vi "Move Drive Motors.vi"(9 "Pneumatics In":T2={"CompressorDevRef"={"DevStatus"={"status"=FALSE, "code"=0, "source"=""}, "Pneumatics Control Module"=0}, "High and Low Gear DoubleSolenoidDevRef"={"DevStatus"={"status"=FALSE, "code"=0, "source"=""}, "Pneumatics Control Module"=0, "Forward Solenoid Channel"=enum."Invalid", "Reverse Solenoid Channel"=enum."Invalid"}, "PTO SolenoidDevRef"={"DevStatus"={"status"=FALSE, "code"=0, "source"=""}, "Pneumatics Control Module"=0, "Forward Solenoid Channel"=enum."Invalid", "Reverse Solenoid Channel"=enum."Invalid"}, "Hang Pin SolenoidDevRef"={"DevStatus"={"status"=FALSE, "code"=0, "source"=""}, "Pneumatics Control Module"=0, "Forward Solenoid Channel"=enum."Invalid", "Reverse Solenoid Channel"=enum."Invalid"}}, 11 "RobotDriveDevRef":T6={"DevStatus"={"status"=FALSE, "code"=0, "source"=""}, "Motors[]"=[], "Square Inputs"=FALSE, "Max Output"=1.0}) -> (1 "Pneumatics Out":T2={"CompressorDevRef"={"DevStatus"={"status"=FALSE, "code"=0, "source"=""}, "Pneumatics Control Module"=0}, "High and Low Gear DoubleSolenoidDevRef"={"DevStatus"={"status"=FALSE, "code"=0, "source"=""}, "Pneumatics Control Module"=0, "Forward Solenoid Channel"=enum."Invalid", "Reverse Solenoid Channel"=enum."Invalid"}, "PTO SolenoidDevRef"={"DevStatus"={"status"=FALSE, "code"=0, "source"=""}, "Pneumatics Control Module"=0, "Forward Solenoid Channel"=enum."Invalid", "Reverse Solenoid Channel"=enum."Invalid"}, "Hang Pin SolenoidDevRef"={"DevStatus"={"status"=FALSE, "code"=0, "source"=""}, "Pneumatics Control Module"=0, "Forward Solenoid Channel"=enum."Invalid", "Reverse Solenoid Channel"=enum."Invalid"}}, 3 "RobotDriveDevRef 2":T6={"DevStatus"={"status"=FALSE, "code"=0, "source"=""}, "Motors[]"=[], "Square Inputs"=FALSE, "Max Output"=1.0})   [LabVIEW 2015]
uses:
  <vilib>/Rock Robotics/WPI/RobotDrive/WPI_RobotDriveDevRef.ctl
  <vilib>/Rock Robotics/WPI/MotorControl/WPI_MotorControlDeviceRef.ctl
  <vilib>/Rock Robotics/WPI/MotorControl/WPI_MotorControlType.ctl
  <vilib>/Rock Robotics/SystemInterfaces/DIO/FPGA_DIOPWMChannel.ctl
  <vilib>/Rock Robotics/WPI/PWM/WPI_PWMDeadband.ctl
  <vilib>/Rock Robotics/WPI/CAN/Jaguar/SubVIs/WPI_CANJaguar_ControlMode.ctl
  <vilib>/Rock Robotics/WPI/CAN/TalonSRX/WPI_CANTalonSRX_APIControlMode.ctl
  Pnematics.ctl
  <vilib>/Rock Robotics/WPI/Compressor/WPI_CompressorDevRef.ctl
  <vilib>/Rock Robotics/WPI/Solenoid/WPI_SolenoidDevRef.ctl
  <vilib>/Rock Robotics/WPI/Solenoid/WPI_SolenoidChannel.ctl
  <vilib>/Rock Robotics/WPI/Solenoid/WPI_SolenoidValue.ctl
  Robot Values.vi
  <vilib>/Rock Robotics/WPI/Solenoid/WPI_SolenoidSetEnum.vi
  <vilib>/Rock Robotics/Network Tables/NT Write String.vi
panel:
  in  "Low":T1=enum."Forward"
  in  "High":T1=enum."Reverse"
  in  "Limits":cluster{"\"Upper\"":dbl, "\"Lower\"":dbl}={"\"Upper\""=1.0, "\"Lower\""=0.1}
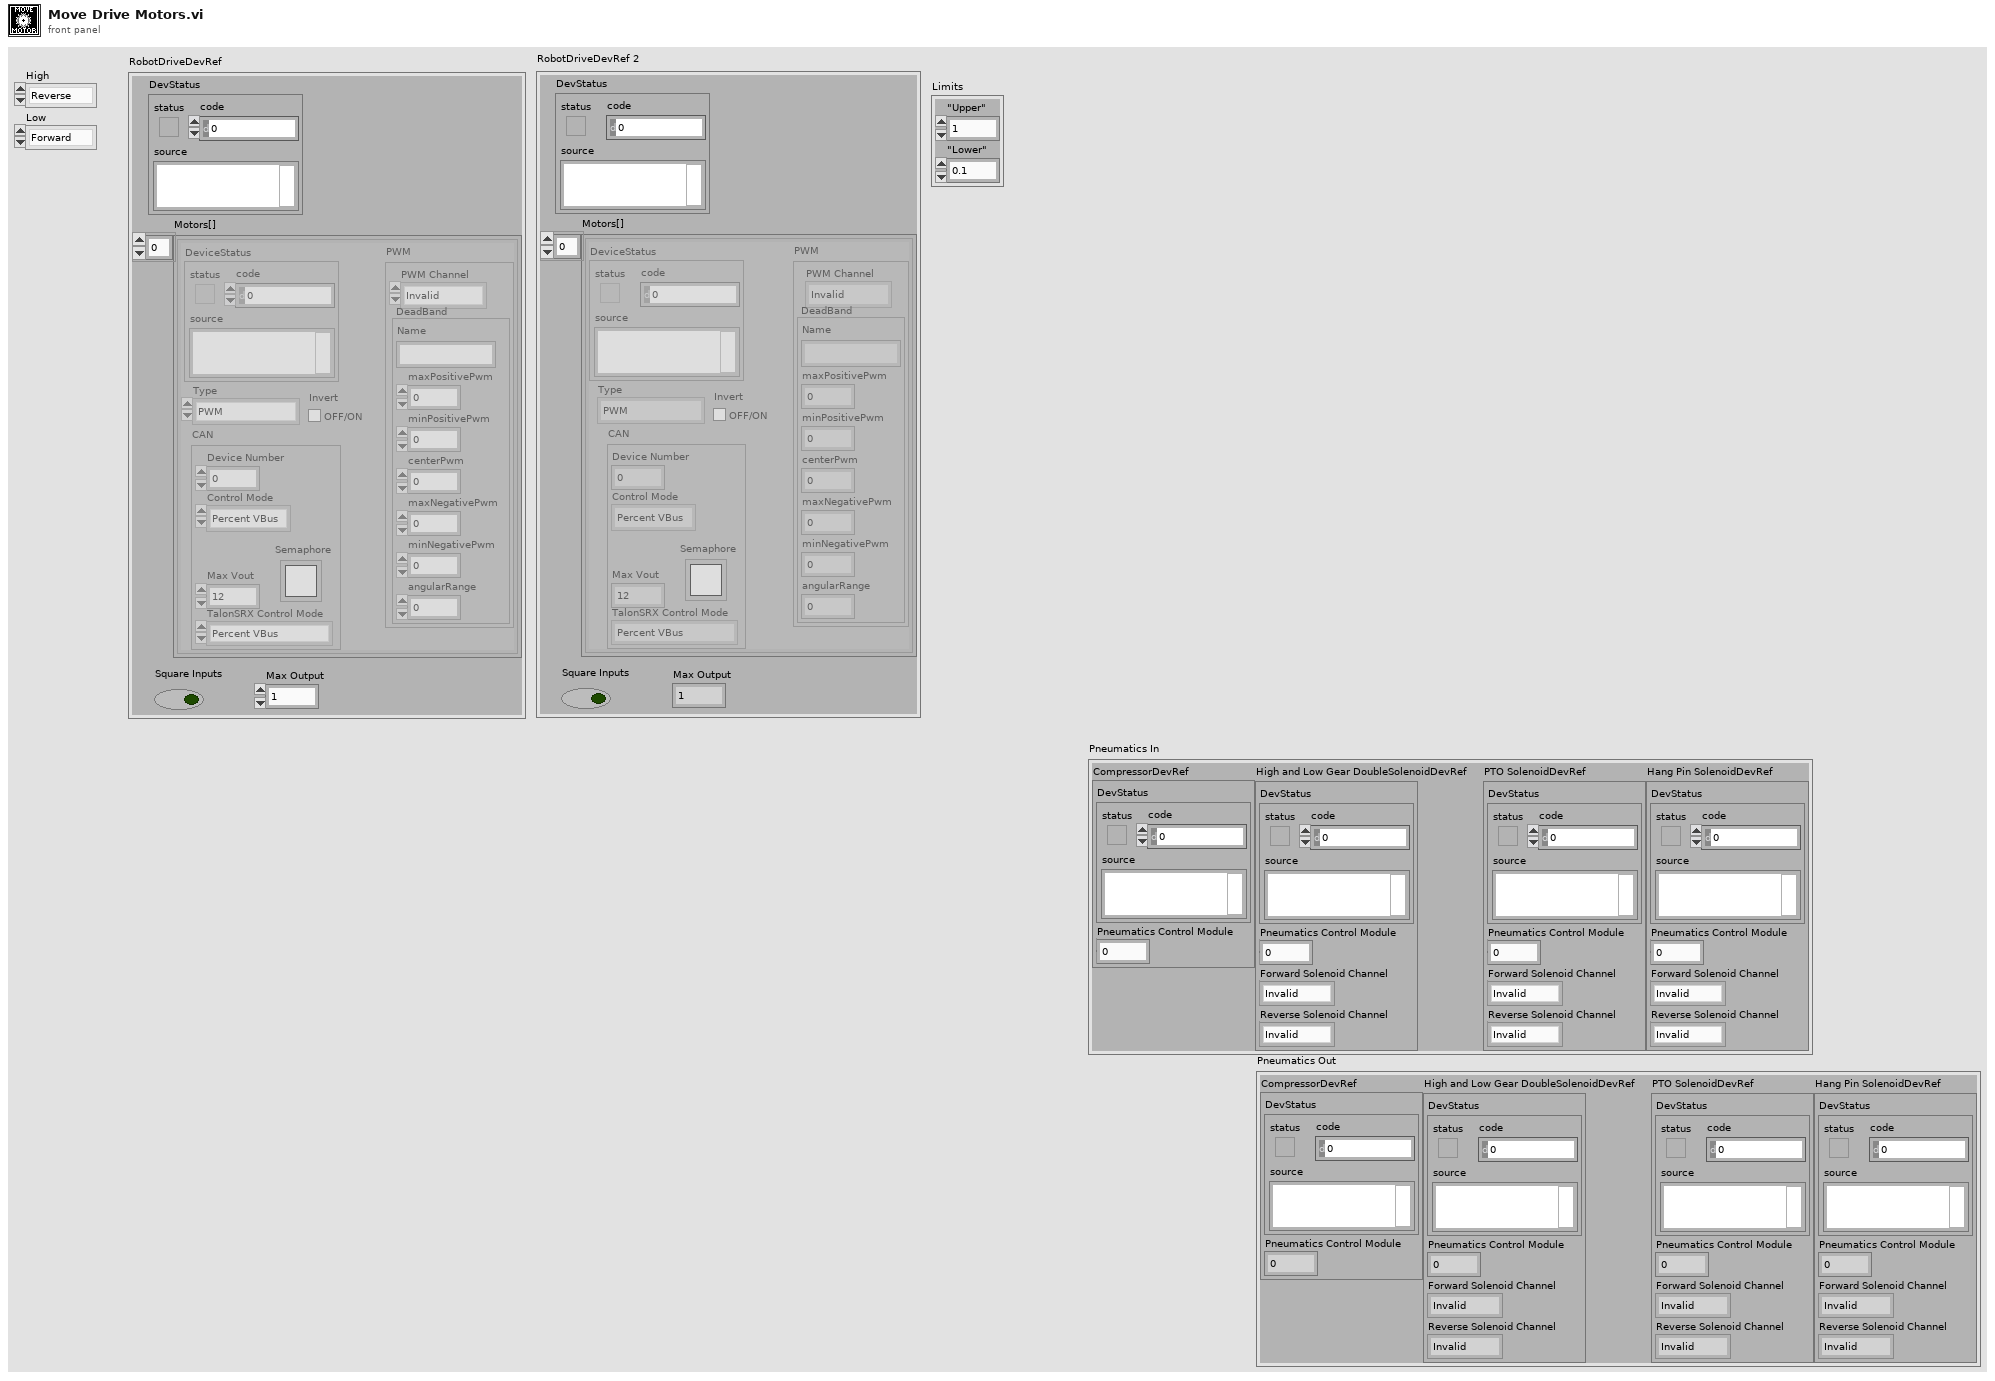
[diagram p1: front panel]
types:
  T1 = typedef "WPI_SolenoidValue.ctl" = enum16{"Off", "On", "Forward", "Reverse"}
  T2 = typedef "Pnematics.ctl" = cluster{"CompressorDevRef":T3, "High and Low Gear DoubleSolenoidDevRef":T4, "PTO SolenoidDevRef":T4, "Hang Pin SolenoidDevRef":T4}
  T3 = typedef "WPI_CompressorDevRef.ctl" = cluster{"DevStatus":errorcluster, "Pneumatics Control Module":u8}
  T4 = typedef "WPI_SolenoidDevRef.ctl" = cluster{"DevStatus":errorcluster, "Pneumatics Control Module":u8, "Forward Solenoid Channel":T5, "Reverse Solenoid Channel":T5}
  T5 = typedef "WPI_SolenoidChannel.ctl" = enum8{"Solenoid 0", "Solenoid 1", "Solenoid 2", "Solenoid 3", "Solenoid 4", "Solenoid 5", "Solenoid 6", "Solenoid 7", "Invalid"}
  T6 = typedef "WPI_RobotDriveDevRef.ctl" = cluster{"DevStatus":errorcluster, "Motors[]":T7[], "Square Inputs":bool, "Max Output":dbl}
  T7 = typedef "WPI_MotorControlDeviceRef.ctl" = cluster{"DeviceStatus":errorcluster, "Type":T8, "PWM":cluster{"PWM Channel":T9, "DeadBand":T10}, "CAN":cluster{"Device Number":u8, "Control Mode":T11, "Semaphore":T12, "Max Vout":dbl, "TalonSRX Control Mode":T13}, "Invert":bool}
  T8 = typedef "WPI_MotorControlType.ctl" = enum16{"PWM", "CAN", "CANTalonSRX"}
  T9 = typedef "FPGA_DIOPWMChannel.ctl" = enum8{"PWM 0", "PWM 1", "PWM 2", "PWM 3", "PWM 4", "PWM 5", "PWM 6", "PWM 7", "PWM 8", "PWM 9", "PWM MXP 0", "PWM MXP 1", "PWM MXP 2", "PWM MXP 3", "PWM MXP 4", "PWM MXP 5", "PWM MXP 6", "PWM MXP 7", "PWM MXP 8", "PWM MXP 9", "Invalid"}
  T10 = typedef "WPI_PWMDeadband.ctl" = cluster{"Name":string, "maxPositivePwm":i32, "minPositivePwm":i32, "centerPwm":i32, "maxNegativePwm":i32, "minNegativePwm":i32, "angularRange":u16}
  T11 = typedef "WPI_CANJaguar_ControlMode.ctl" = enum8{"Percent VBus", "Current", "Speed", "Position", "Voltage"}
  T12 = typedef "Semaphore RefNum" = refnum<k1>
  T13 = typedef "WPI_CANTalonSRX_APIControlMode.ctl" = enum8{"Percent VBus", "Speed", "Position", "Slave", "Unchanged / Invalid", "Voltage Compensation", "Current", "Motion Profile"}
  T14 = typedef "Robot Values.ctl" = cluster{"Drive Motors":cluster{"Left Motor Value":dbl, "Right Motor Value":dbl, "Left Motor Encoder":dbl, "Right Motor Encoder":dbl, "High/Low Gear":bool}, "Sensors":cluster{"Gyro Angle":dbl, "Photoeye":bool, "Ultrasonic Range":dbl, "Shooter Speed Encoder":dbl, "Accelerometer Value":dbl, "Flashlight":bool, "Target Distance":dbl, "Target X Value":dbl}, "Arms":cluster{"Desired Arm Position":dbl, "Left Arm Encoder":dbl, "Right Arm Encoder":dbl, "Left Arm Lower Limit":bool, "Right Arm Lower Limit":bool, "Initialize Arm Position?":bool}, "Acquisition and Scoring":cluster{"Acquiring?":bool, "Current Speed":dbl, "Setpoint Speed":dbl, "Prep Wheels":bool, "Shoot":bool, "Low Eject":bool}, "Hanging":cluster{"Pivot Arms":dbl, "PTO":bool, "Left Pivot Encoder":dbl, "Right Pivot Encoder":dbl, "Hanging Pin":bool}}
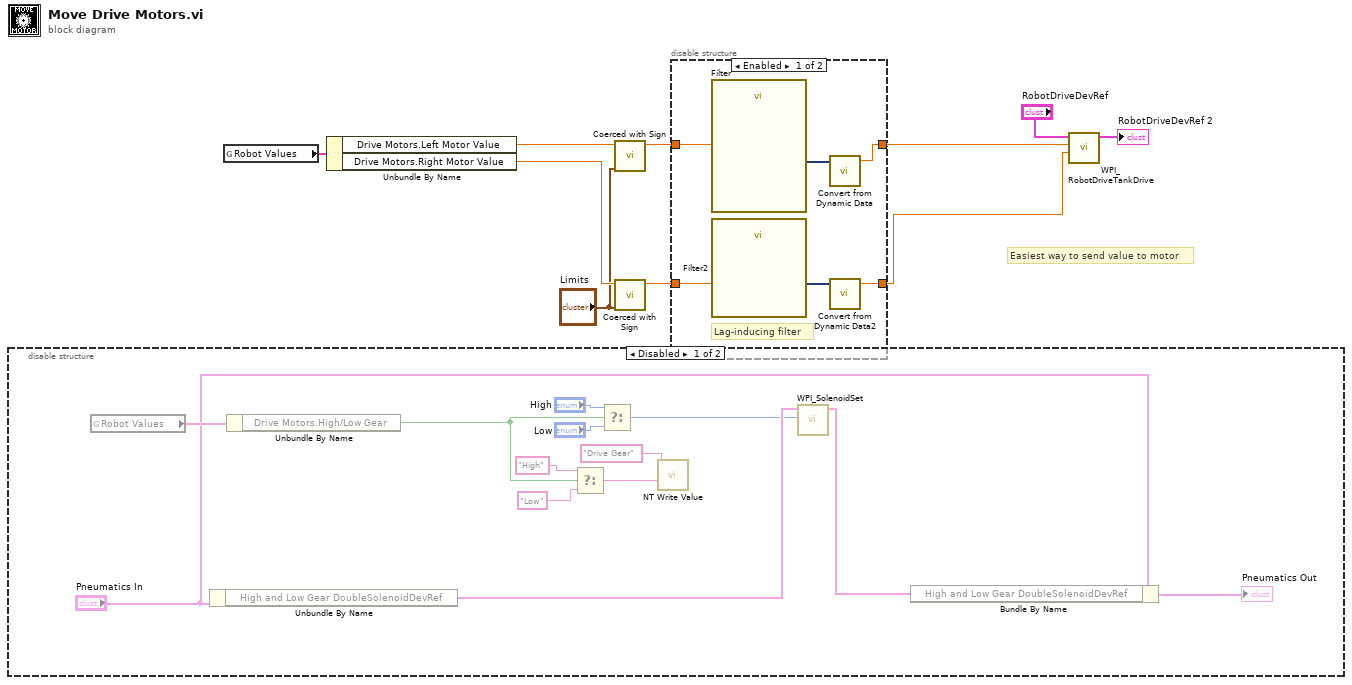
[diagram p0: block diagram]
diagram:
  # "Easiest way to send value to motor"
  n1 = disable-structure shown="Disabled" {
    frame Disabled {
      n2 = global read "Robot Values.vi" "Robot Values"() -> (w23:T14)
      n3 = Unbundle By Name("Pneumatics In") -> ("High and Low Gear DoubleSolenoidDevRef"=w20:T4)
      n4 = Unbundle By Name(w23) -> ("Drive Motors.High/Low Gear"=w17:bool)
      n5 = Select(t="High", s=w17, f="Low") -> (s? t:f=w14:string)
      n6 = Select(t="High", s=w17, f="Low") -> (s? t:f=w19:T1)
      n7 = call-poly <vilib>:"NT Write Value.vi"("String"=w14, "Name"="Drive Gear") -> ()  [unwired: 9 in, 1 out]
      n8 = call-poly <vilib>:"WPI_SolenoidSet.vi"("Value"=w19, "SolenoidDevRef"=w20) -> ("SolenoidDevRef"=w18:T4)  [unwired: 8 in, 1 out]
      n9 = Bundle By Name(cluster="Pneumatics In", "High and Low Gear DoubleSolenoidDevRef"=w18) -> (→"Pneumatics Out":T2)
    }
    frame Enabled {
    }
  }
  n10 = global read "Robot Values.vi" "Robot Values"() -> (w10:T14)
  n11 = Unbundle By Name(w10) -> ("Drive Motors.Left Motor Value"=w7:dbl, "Drive Motors.Right Motor Value"=w6:dbl)
  n12 = call "Coerced with Sign.vi"("Input"=w7, "Limits"="Limits") -> ("Coerced"=w5:dbl)  [unwired: 7 in, 1 out]
  n13 = call "Coerced with Sign.vi"("Input"=w6, "Limits"="Limits") -> ("Coerced"=w4:dbl)  [unwired: 7 in, 1 out]
  n14 = disable-structure shown="Enabled" {
    disable-tunnel: w5 -> [w29 w31]
    disable-tunnel: [w26 w31] -> w2
    disable-tunnel: w4 -> [w28 w30]
    disable-tunnel: [w24 w30] -> w1
    frame Enabled {
      # "Lag-inducing filter"
      n15 = call "Filter"("Signal"=w29) -> ("Filtered Signal"=w27:dynamicdata)  [unwired: 9 in, 1 out]
      n16 = call "Filter2"("Signal"=w28) -> ("Filtered Signal"=w25:dynamicdata)  [unwired: 9 in, 1 out]
      n17 = call "Convert from Dynamic Data"("Dynamic Data Type"=w27) -> ("Scalar"=w26:dbl)  [unwired: 3 in]
      n18 = call "Convert from Dynamic Data2"("Dynamic Data Type"=w25) -> ("Scalar"=w24:dbl)  [unwired: 3 in]
    }
    frame Disabled {
    }
  }
  n19 = call <vilib>:"WPI_RobotDriveTankDrive.vi"("Right axis value"=w1, "Left axis value"=w2, "RobotDriveDevRef"="RobotDriveDevRef") -> ("RobotDriveDevRef"=→"RobotDriveDevRef 2":T6)  [unwired: 6 in, 2 out]
